vi "DefendAreaTacticCheckStateChange.vi"(8 "error in (no error)":errorcluster, 10 "Game":refnum<class "Game.lvclass">, 11 "DefendAreaTactic in":refnum<class "DefendAreaTactic.lvclass">) -> (0 "error out":errorcluster, 2 "States":T1=enum."BlockPossibleShot", 3 "DefendAreaTactic out":refnum<class "DefendAreaTactic.lvclass">)   [LabVIEW 2024, in "DefendAreaTactic.lvclass"]
uses:
  DefendAreaTactic.lvclass
  Game_class/Game.lvclass
  DefendAreaTacticStates.ctl
  Game_class/Game.lvclass/Game.ctl
  Events_class/Events.lvclass/Events.ctl
  Ball_class/Ball.lvclass/Ball.ctl
  Game_class/Read FieldRef.vi
  Game_class/Read EventsRef.vi
  Game_class/Read BallRef.vi
  Ball_class/Read velocityNorm.vi
  Events_class/Read ball_inside_our_goalie_area.vi
  <vilib>/Analysis/_algsub.llb/Vector Norm.vi
  <vilib>/Analysis/_algsub.llb/Real Vector Norm.vi
  Field_class/Field.lvclass
  Events_class/Events.lvclass
  Ball_class/Ball.lvclass
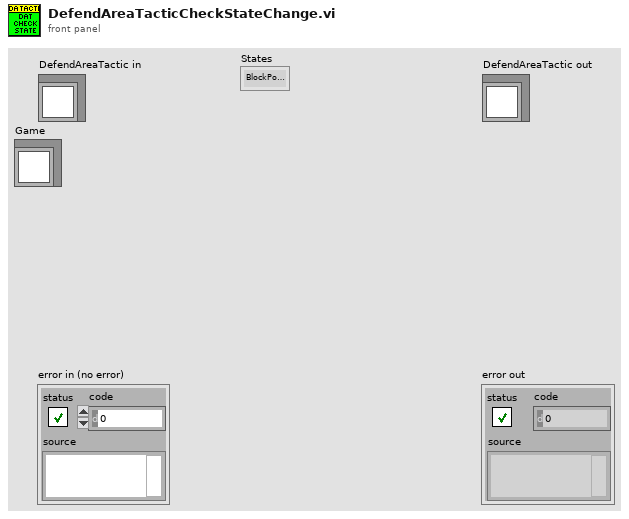
[diagram p1: front panel]
types:
  T1 = typedef "DefendAreaTactic.lvclass/DefendAreaTacticStates.ctl" = enum16{"BlockShot", "BlockPossibleShot", "CoverOneTouchShot", "BallInKeeperArea", "Exit"}
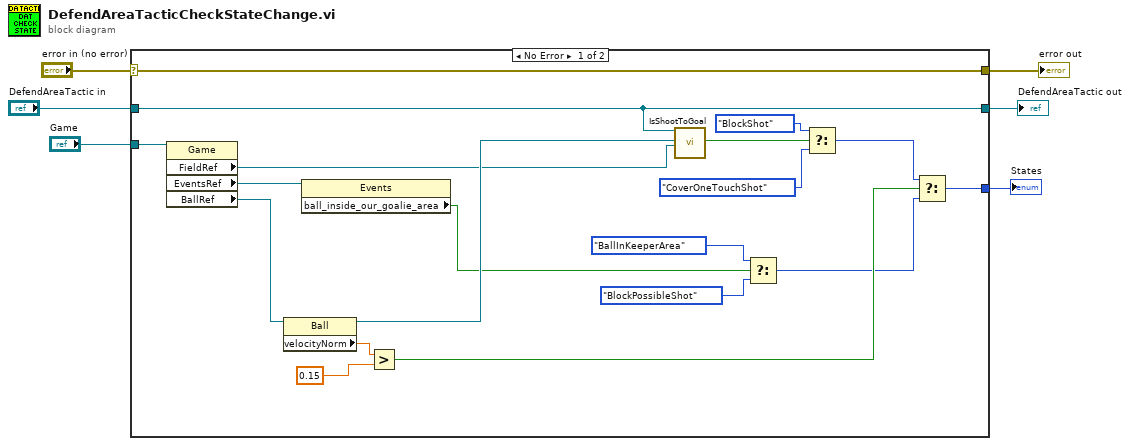
[diagram p0: block diagram]
diagram:
  n1 = case shown="No Error" "error in (no error)" {
    selector: "error in (no error)" -> [w25 w27]
    tunnel: [w25 w27] -> w5
    tunnel: [w17 w26] -> w3
    tunnel: "DefendAreaTactic in" -> [w17 w26]
    tunnel: "Game" -> [w24 _]
    tunnel: [w22 _] -> w1
    frame No Error {
      n2 = property class="Game"(reference=w24) -> ("FieldRef"=w15:refnum<class "Field.lvclass">, "EventsRef"=w8:refnum<class "Events.lvclass">, "BallRef"=w23:refnum<class "Ball.lvclass">)  [unwired: 1 in, 2 out]
      n3 = property class="Ball"(reference=w23) -> (reference out=w16:refnum<class "Ball.lvclass">, "velocityNorm"=w21:dbl)  [unwired: 1 in, 1 out]
      n4 = property class="Events"(reference=w8) -> ("ball_inside_our_goalie_area"=w7:bool)  [unwired: 1 in, 2 out]
      n5 = Greater?(x=w21, y=0.15) -> (0:w20:bool)
      n6 = call "IsShootToGoal.vi"("object in"=w17, "Ball"=w16, "Field"=w15) -> ("IsShoot"=w14:bool)  [unwired: 13 in, 3 out]
      n7 = Select(t=DefendAreaTacticStates."BallInKeeperArea" ("States"), s=w7, f=DefendAreaTacticStates."BlockPossibleShot" ("States")) -> (s? t:f=w13:T1)
      n8 = Select(t=DefendAreaTacticStates."BlockShot" ("States"), s=w14, f=DefendAreaTacticStates."CoverOneTouchShot" ("States")) -> (s? t:f=w19:T1)
      n9 = Select(t=w19, s=w20, f=w13) -> (s? t:f=w22:T1)
    }
    frame Error {
    }
  }
  "error out" <- w5
  "DefendAreaTactic out" <- w3
  "States" <- w1
